vi "Export Log File.vi"(8 "error in":errorcluster, 11 "File Data":string[](array[string])) -> (0 "error out":errorcluster)   [LabVIEW 2020, in "SECS Bridge.lvlib"]
uses:
  SECS Bridge.lvlib
  <vilib>/DATA AHEAD/XLR8/functions/Workbook/Open Create Workbook XLSX.vi
  <vilib>/DATA AHEAD/XLR8/subs/Polymorphic VIs Sources/(Clear Sheet and) Write Area - String.vi
  <vilib>/DATA AHEAD/XLR8/XLR8.lvlib
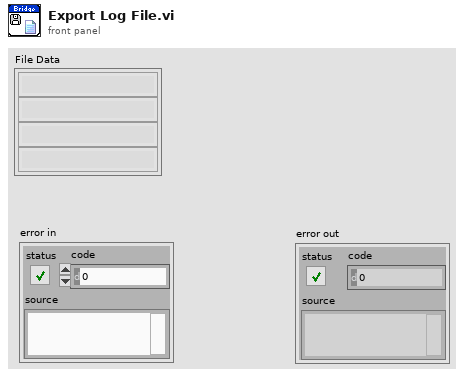
[diagram p1: front panel]
types:
  T1 = typedef "XLR8.lvlib/XLR8_Ref.ctl" = cluster{"WBK":refnum<k24>, "CurSheet":refnum<k24>, "File":refnum<k24>, "file path":string, "sheet":string, "Sheets":refnum<k24>[], "IsXML":bool, "Policy":i32}
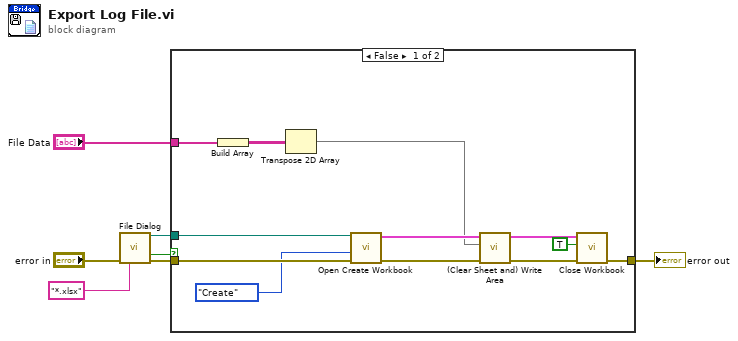
[diagram p0: block diagram]
diagram:
  n1 = call "File Dialog"("error in"="error in", "pattern (all files)"="*.xlsx") -> ("selected path"=w3:path, "cancelled"=w4:bool, "error out"=w5:errorcluster)  [unwired: 10 in, 1 out]
  n2 = case shown="False" w4 {
    tunnel: w5 -> [w19 _]
    tunnel: w3 -> [w18 _]
    tunnel: "File Data" -> [w14 _]
    tunnel: [w8 _] -> w1
    frame False {
      n3 = Build Array(w14) -> (w13:string[][])
      n4 = Transpose 2D Array(2D array=w13) -> (transposed array=w12:string[][])
      n5 = call-poly <vilib>:"Open Create Workbook.vi"("error in"=w19, "Open or Create"=enum16{"Create", "Open"}."Create", "Workbook Path"=w18) -> ("error out"=w16:errorcluster, "Refs Out"=w15:T1)  [unwired: 7 in]
      n6 = call-poly <vilib>:"(Clear Sheet and) Write Area.vi"("error in"=w16, "Array"=w12, "Refs In"=w15) -> ("error out"=w10:errorcluster, "Refs Out"=w11:T1)  [unwired: 7 in]
      n7 = call <vilib>:"Close Workbook.vi"("error in"=w10, "Save File? (F)"=TRUE, "Refs In"=w11) -> ("error out"=w8:errorcluster)  [unwired: 7 in, 1 out]
    }
    frame True {
    }
  }
  "error out" <- w1
